vi "Pre-Alpha.vi"() -> ()   [LabVIEW 2010]
panel:
  in  "File Type":enum16{"PNG", "JPEG", "BMP"}(ring)
  out "2D Picture":picture
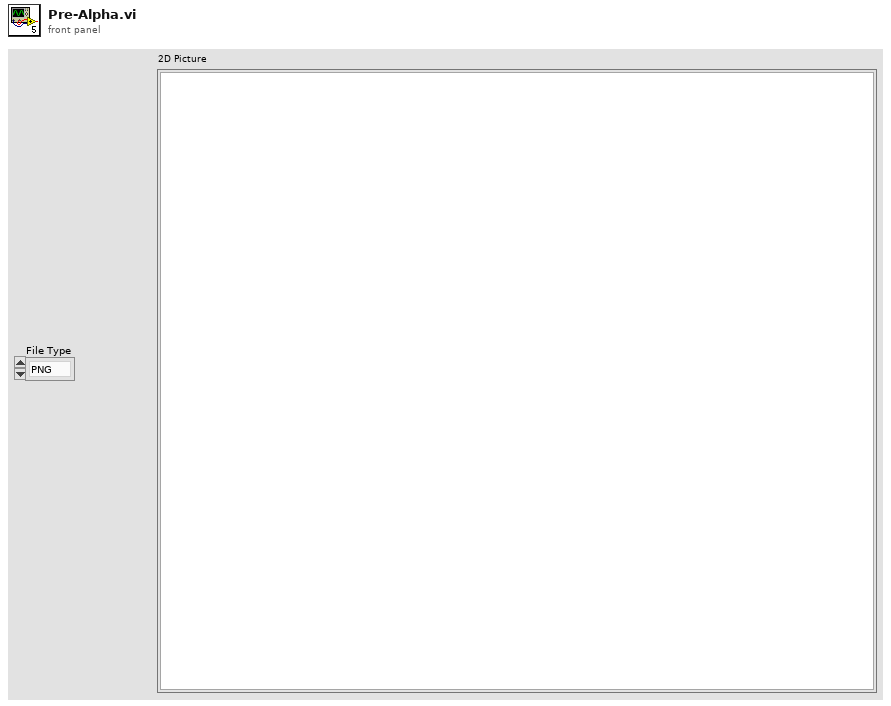
[diagram p1: front panel]
types:
  T1 = typedef "imagedata.ctl" = cluster{"image type":i32, "image depth":i32, "image":u8[], "mask":u8[], "colors":u32[], "Rectangle":cluster{"left":i16, "top":i16, "right":i16, "bottom":i16}}
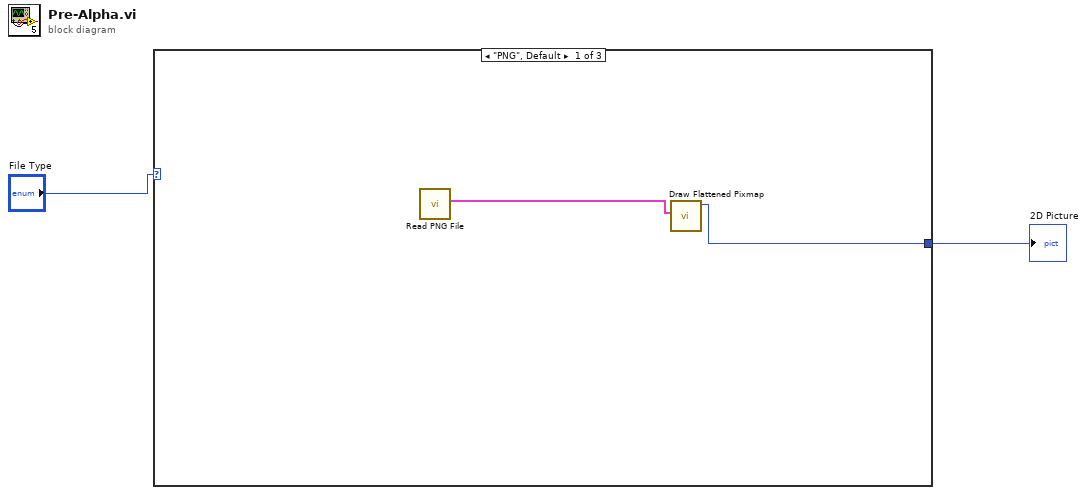
[diagram p0: block diagram]
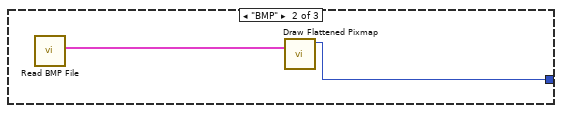
[diagram p2: hidden frame]
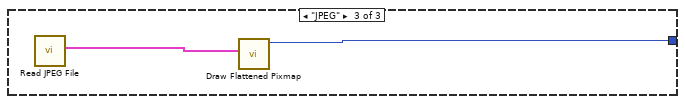
[diagram p3: hidden frame]
diagram:
  n1 = case shown="\"PNG\", Default" "File Type" {
    tunnel: [w3 w5 w7] -> w2
    frame "PNG", Default {
      n2 = call <vilib>:"Read PNG File.vi"() -> ("image data"=w4:T1)  [unwired: 9 in, 2 out]
      n3 = call <vilib>:"Draw Flattened Pixmap.vi"("image data"=w4) -> ("new picture"=w3:picture)  [unwired: 8 in]
    }
    frame "BMP" {
      n4 = call <vilib>:"Read BMP File.vi"() -> ("image data"=w6:T1)  [unwired: 9 in, 2 out]
      n5 = call <vilib>:"Draw Flattened Pixmap.vi"("image data"=w6) -> ("new picture"=w5:picture)  [unwired: 8 in]
    }
    frame "JPEG" {
      n6 = call <vilib>:"Read JPEG File.vi"() -> ("image data"=w8:T1)  [unwired: 9 in, 2 out]
      n7 = call <vilib>:"Draw Flattened Pixmap.vi"("image data"=w8) -> ("new picture"=w7:picture)  [unwired: 8 in]
    }
  }
  "2D Picture" <- w2
